vi "DP_NextStep.vi"(8 "error in (no error)":errorcluster, 10 "DAtoDP":T1={"Accessibility"={"Command"=enum."End", "Error?"=FALSE, "Stop"=FALSE, "StopPomiar"=FALSE, "Name"="", "FilesPath"=path "", "ErrorHandler"={"Threads"=enum."Acquisistion", "ClearError"=FALSE, "Error Out "={"status"=FALSE, "code"=0, "source"=""}, "Error"=FALSE}, "Fs"=0.0}, "RawData"=[], "Counter"=0, "Fs"=0.0}, 11 "PreviousStep":T5) -> (0 "error out":errorcluster, 3 "NextStep":T5)   [LabVIEW 2019]
uses:
  TypeDef/#TypeDef_EnumOp_DataProcessing.ctl
  TypeDef/#TypeDef_PropFromDAtoDP.ctl
  Communication/TypeDef/#TypeDef_FromPCtoMR.ctl
  Communication/TypeDef/#TypeDef_Command.ctl
  Communication/TypeDef/#TypeDef_ErrorHandler_prop.ctl
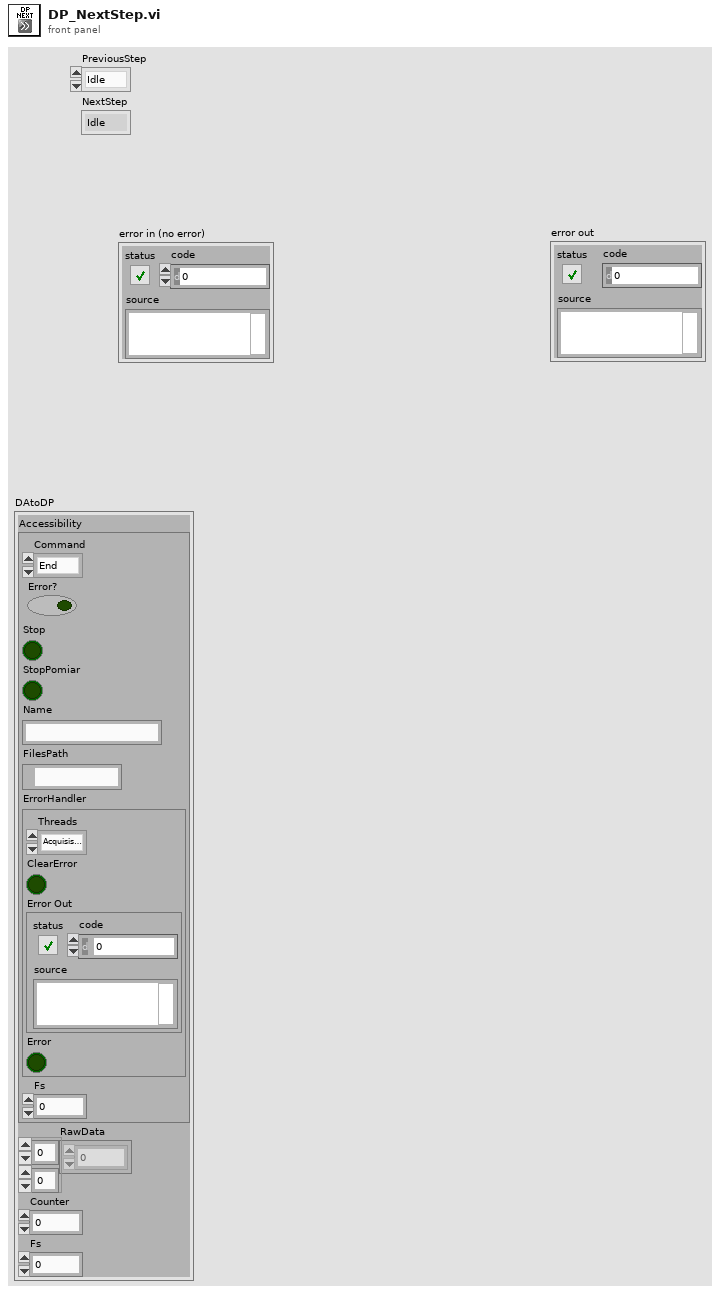
[diagram p1: front panel]
types:
  T1 = typedef "#TypeDef_PropFromDAtoDP.ctl" = cluster{"Accessibility":T2, "RawData":dbl[][], "Counter":i32, "Fs":dbl}
  T2 = typedef "#TypeDef_FromPCtoMR.ctl" = cluster{"Command":T3, "Error?":bool, "Stop":bool, "StopPomiar":bool, "Name":string, "FilesPath":path, "ErrorHandler":T4, "Fs":dbl}
  T3 = typedef "#TypeDef_Command.ctl" = enum16{"Start", "End"}
  T4 = typedef "#TypeDef_ErrorHandler_prop.ctl" = cluster{"Threads":enum16{"Acquisistion", "Data Operation", "Save File"}, "ClearError":bool, "Error Out ":errorcluster, "Error":bool}
  T5 = typedef "#TypeDef_EnumOp_DataProcessing.ctl" = enum16{"Idle", "Init", "Operations", "End", "Error_Shutdown", "ClearError"}
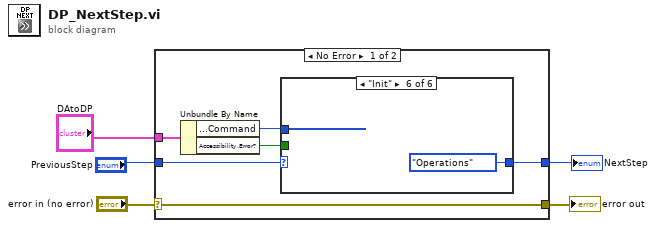
[diagram p0: block diagram]
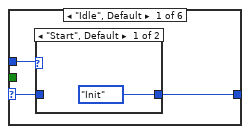
[diagram p2: hidden frame]
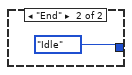
[diagram p3: hidden frame]
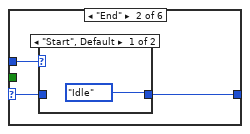
[diagram p4: hidden frame]
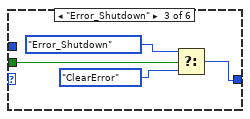
[diagram p6: hidden frame]
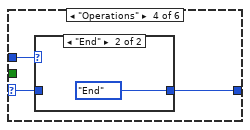
[diagram p7: hidden frame]
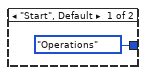
[diagram p8: hidden frame]
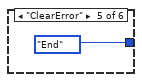
[diagram p9: hidden frame]
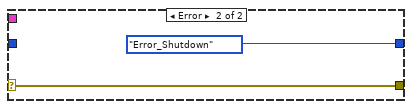
[diagram p10: hidden frame]
diagram:
  n1 = case shown="No Error" "error in (no error)" {
    selector: "error in (no error)" -> [w10 w33]
    tunnel: [w10 w33] -> w5
    tunnel: [w6 #TypeDef_EnumOp_DataProcessing."Error_Shutdown" ("EnumOp_DataAcquisition")] -> w2
    tunnel: "DAtoDP" -> [w9 _]
    tunnel: "PreviousStep" -> [w8 _]
    frame No Error {
      n2 = Unbundle By Name(w9) -> ("Accessibility.Command"=w11:T3, "Accessibility.Error?"=w7:bool)
      n3 = case shown="\"Init\"" w8 {
        selector: w8 -> [w13 w18 _ w26 _ _]
        tunnel: w11 -> [w14 w19 _ w25 _ _]
        tunnel: [w12 w17 w23 w27 #TypeDef_EnumOp_DataProcessing."End" ("EnumOp_DataAcquisition") #TypeDef_EnumOp_DataProcessing."Operations" ("EnumOp_DataAcquisition")] -> w6
        tunnel: w7 -> [_ _ w24 _ _ _]
        frame "Idle", Default {
          n4 = case shown="\"Start\", Default" w14 {
            tunnel: [#TypeDef_EnumOp_DataProcessing."Init" ("EnumOp_DataAcquisition") #TypeDef_EnumOp_DataProcessing."Idle" ("EnumOp_DataAcquisition")] -> w12
            tunnel: w13 -> [_ _]
            frame "Start", Default {
            }
            frame "End" {
            }
          }
        }
        frame "End" {
          n5 = case shown="\"Start\", Default" w19 {
            tunnel: w18 -> [_ _]
            tunnel: [#TypeDef_EnumOp_DataProcessing."Idle" ("EnumOp_DataAcquisition") _] -> w17
            frame "Start", Default {
            }
            frame "End" {
            }
          }
        }
        frame "Error_Shutdown" {
          n6 = Select(t=#TypeDef_EnumOp_DataProcessing."Error_Shutdown" ("EnumOp_DataAcquisition"), s=w24, f=#TypeDef_EnumOp_DataProcessing."ClearError" ("EnumOp_DataAcquisition")) -> (s? t:f=w23:T5)
        }
        frame "Operations" {
          n7 = case shown="\"End\"" w25 {
            tunnel: [#TypeDef_EnumOp_DataProcessing."Operations" ("EnumOp_DataAcquisition") #TypeDef_EnumOp_DataProcessing."End" ("EnumOp_DataAcquisition")] -> w27
            tunnel: w26 -> [_ _]
            frame "Start", Default {
            }
            frame "End" {
            }
          }
        }
        frame "ClearError" {
        }
        frame "Init" {
        }
      }
    }
    frame Error {
    }
  }
  "error out" <- w5
  "NextStep" <- w2
